vi "RSZVB Get TDIF Source Power Mode.vi"(8 "error in (no error)":errorcluster {"code" format="%.0x"}, 10 "Channel (1)":i32=1, 11 "VISA session":refnum<visa-resource-name>) -> (0 "error out":errorcluster {"code" format="%.0x"}, 2 "Source Power Mode":i32, 3 "dup VISA session":refnum<visa-resource-name>)   [LabVIEW 2011]
doc: "This VI returns source power mode. \n\nNote(s):\n\n(1) This VI is available only with option R&S ZVA-K6 and ZVT instrument.\n\nRemote-control command(s):\nSOURce<Ch>:TDIF:WAVes?"
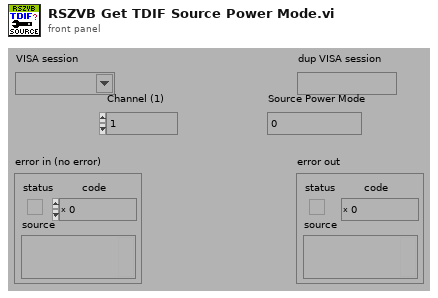
[diagram p1: front panel]
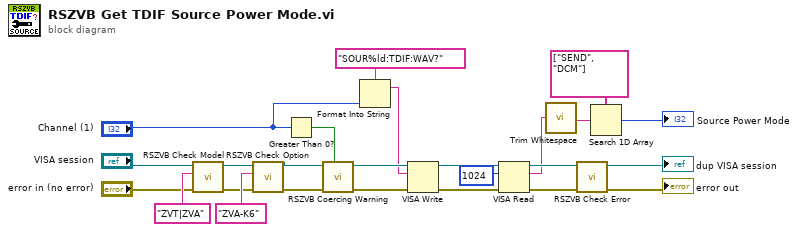
[diagram p0: block diagram]
diagram:
  n1 = call "RSZVB Check Model.vi"("error in (no error)"="error in (no error)", "Model"="ZVT|ZVA" ("Options"), "VISA session"="VISA session") -> ("error out"=w10:errorcluster, "dup VISA session"=w11:refnum<visa-resource-name>)  [unwired: 7 in]
  n2 = call "RSZVB Check Option.vi"("error in (no error)"=w10, "Options"="ZVA-K6", "VISA session"=w11) -> ("error out"=w8:errorcluster, "dup VISA session"=w7:refnum<visa-resource-name>)  [unwired: 7 in]
  n3 = Greater Than 0?(x="Channel (1)") -> (x > 0?=w16:bool)
  n4 = call "RSZVB Coercing Warning.vi"("In Range?"=w16, "error in (no error)"=w8, "VISA session"=w7) -> ("error out"=w23:errorcluster, "dup VISA session"=w24:refnum<visa-resource-name>)  [unwired: 7 in]
  n5 = Format Into String(format string="SOUR%ld:TDIF:WAV?", "Channel (1)") -> (resulting string=w22:string)  [unwired: 2 in, 1 out]
  n6 = VISA Write(VISA resource name=w24, write buffer=w22, error in (no error)=w23) -> (VISA resource name out=w19:refnum<visa-resource-name>, error out=w21:errorcluster)  [unwired: 1 out]
  n7 = VISA Read(VISA resource name=w19, byte count=u32 1024 ("byte count (0)"), error in (no error)=w21) -> (VISA resource name out=w18:refnum<visa-resource-name>, read buffer=w13:string, error out=w17:errorcluster)  [unwired: 1 out]
  n8 = call <vilib>:"Trim Whitespace.vi"("string"=w13) -> ("trimmed string"=w14:string)  [unwired: 1 in]
  n9 = call "RSZVB Check Error.vi"("error in (no error)"=w17, "VISA session"=w18) -> ("error out"=→"error out":errorcluster, "dup VISA session"=→"dup VISA session":refnum<visa-resource-name>)  [unwired: 8 in]
  n10 = Search 1D Array(1D array=string[] ["SEND", "DCM"] ("array 2"), element=w14) -> (index of element=→"Source Power Mode":i32)  [unwired: 1 in]
